vi "Get Controller Name from IDN.vi"(0 "Identification":string, 5 "error in":errorcluster) -> (14 "Controller Name":T1, 15 "System Name":string, 16 "Full System Name":string, 19 "error out":errorcluster)   [LabVIEW 2020]
doc: "This VI extracts the system name from the *IDN? answer."
uses:
  Controller names.ctl
panel:
  # "This VI extracts the system name from the *IDN? answer."
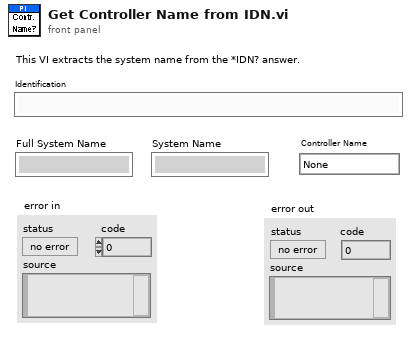
[diagram p1: front panel]
types:
  T1 = typedef "Controller names.ctl" = enum16{"None", "Analog", "C-702", "C-413", "C-414", "C-843", "C-843.PM", "C-844", "C-848", "C-865", "C-866", "C-867", "C-877", "C-880", "C-884", "C-885", "C-886", "C-887", "C-891", "E-135", "E-516", "E-517", "E-518", "E-709", "E-710", "E-712", "E-725", "E-727", "E-753", "E-754", "E-755", "E-761", "E-816", "E-861", "E-870", "E-871", "E-872", "E-873", "E-874", "F-206", "HydraPollux", "M-840", "M-850", "M-8X0", "Mercury", "Mercury_GCS", "PI_GCS2"}
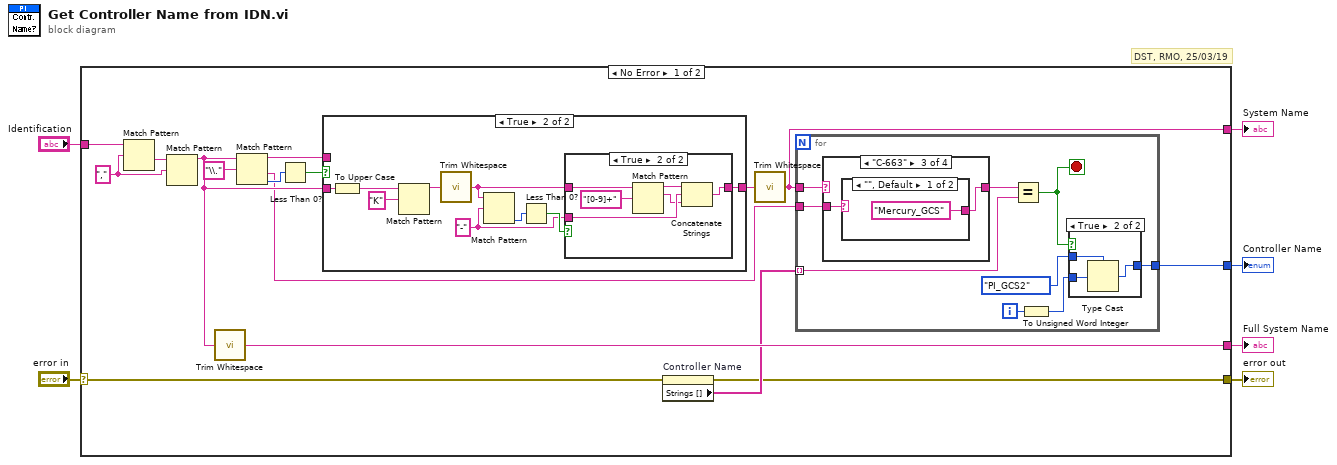
[diagram p0: block diagram]
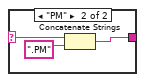
[diagram p4: hidden frame]
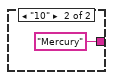
[diagram p5: hidden frame]
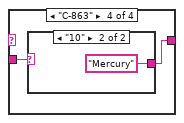
[diagram p6: hidden frame]
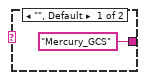
[diagram p7: hidden frame]
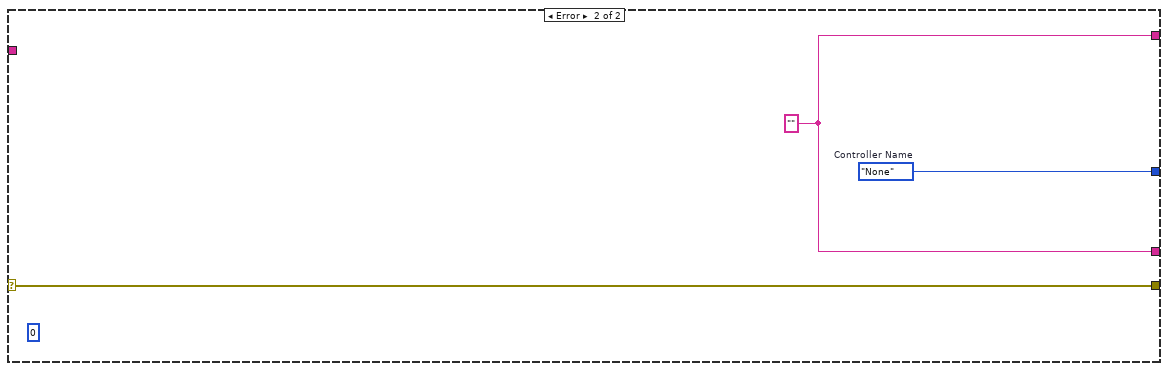
[diagram p11: hidden frame]
diagram:
  # "DST, RMO, 25/03/19"
  n1 = case shown="No Error" "error in" {
    selector: "error in" -> [w10 w70]
    tunnel: "Identification" -> [w22 _]
    tunnel: [w18 w69] -> w5
    tunnel: [w11 w69] -> w4
    tunnel: [w7 w68] -> w3
    tunnel: [w9 w70] -> w1
    frame No Error {
      w21 = "," ("regular expression")
      n2 = Match Pattern(string=w22, regular expression=w21) -> (after substring=w20:string)  [unwired: 4 out]
      n3 = Match Pattern(string=w20, regular expression=w21) -> (before substring=w15:string)  [unwired: 4 out]
      n4 = call "Trim Whitespace.vi"("string"=w15) -> ("trimmed string"=w18:string)  [unwired: 1 in]
      n5 = Match Pattern(string=w15, regular expression="\\.") -> (before substring=w14:string, after substring=w8:string, offset past match=w17:i32)  [unwired: 2 out]
      n6 = Less Than 0?(x=w17) -> (x < 0?=w16:bool)
      n7 = case shown="True" w16 {
        tunnel: w15 -> [_ w60]
        tunnel: w14 -> [w51 _]
        tunnel: [w51 w53] -> w13
        frame False {
        }
        frame True {
          w52 = "-" ("regular expression")
          n8 = To Upper Case(1:w60) -> (0:w59:string)
          n9 = Match Pattern(string=w59, regular expression="K") -> (before substring=w57:string)  [unwired: 4 out]
          n10 = call "Trim Whitespace.vi"("string"=w57) -> ("trimmed string"=w54:string)  [unwired: 1 in]
          n11 = Match Pattern(string=w54, regular expression=w52) -> (offset past match=w56:i32)  [unwired: 4 out]
          n12 = Less Than 0?(x=w56) -> (x < 0?=w55:bool)
          n13 = case shown="True" w55 {
            tunnel: w54 -> [w61 w66]
            tunnel: [w61 w63] -> w53
            tunnel: w52 -> [_ w64]
            frame False {
            }
            frame True {
              n14 = Match Pattern(string=w66, regular expression="[0-9]+") -> (before substring=w65:string, match substring=w62:string)  [unwired: 3 out]
              n15 = Concatenate Strings(w65, w64, w62) -> (w63:string)
            }
          }
        }
      }
      n16 = property on="Controller Name" class="Enum (strict)"(error in=w10) -> (error out=w9:errorcluster, "Strings []"=w12:string[])  [unwired: 1 in, 1 out]
      n17 = call "Trim Whitespace.vi"("string"=w13) -> ("trimmed string"=w11:string)  [unwired: 1 in]
      n18 = for {
        tunnel: w12 -> [w31] mode=indexing
        tunnel: w11 -> [w27]
        tunnel: [w29] -> w7
        tunnel: w8 -> [w25]
        i -> [w30]
        stop <- w28 stop-if-true
        n19 = case shown="\"C-663\"" w27 {
          selector: w27 -> [w32 _ _ _]
          tunnel: [w32 w33 w39 w43] -> w26
          tunnel: w25 -> [_ w34 w40 w44]
          frame "None", Default {
          }
          frame "C-843" {
            n20 = case shown="\"\", Default" w34 {
              selector: w34 -> [w35 w38]
              tunnel: [w35 w36] -> w33
              frame "", Default {
              }
              frame "PM" {
                n21 = Concatenate Strings(w38, ".PM" ("string")) -> (w36:string)
              }
            }
          }
          frame "C-663" {
            n22 = case shown="\"\", Default" w40 {
              tunnel: ["Mercury_GCS" "Mercury"] -> w39
              frame "", Default {
              }
              frame "10" {
              }
            }
          }
          frame "C-863" {
            n23 = case shown="\"10\"" w44 {
              tunnel: ["Mercury_GCS" "Mercury"] -> w43
              frame "", Default {
              }
              frame "10" {
              }
            }
          }
        }
        n24 = Equal?(x=w26, y=w31) -> (x = y?=w28:bool)
        n25 = To Unsigned Word Integer(number=w30) -> (unsigned 16bit integer=w23:u16)
        n26 = case shown="True" w28 {
          tunnel: w23 -> [_ w50]
          tunnel: [w47 w48] -> w29
          tunnel: Controller_names."PI_GCS2" ("Controller Name") -> [w47 w49]
          frame False {
          }
          frame True {
            n27 = Type Cast(type=w49, x=w50) -> (*(type *) &x=w48:T1)
          }
        }
      }
    }
    frame Error {
      w68 = Controller_names."None"  # Controller Name
      (unwired) u16 0
      w69 = ""
    }
  }
  "Controller Name" <- w3
  "Full System Name" <- w5
  "System Name" <- w4
  "error out" <- w1
